vi "Custom Standard.vi"(0 "IL Enable":bool=TRUE, 5 "RL Enable":bool=TRUE) -> (7 "Output Custom":T1)   [LabVIEW 2017]
panel:
  in  "Min RL to Pass (dB)":dbl format="%#.2g"
  in  "Max IL to Pass (dB)":dbl=99.0 format="%.2g"
  in  "End Process":bool
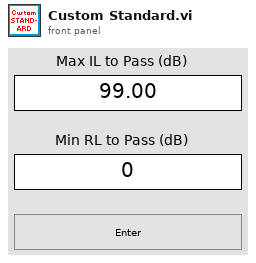
[diagram p1: front panel]
types:
  T1 = cluster{"Standard Name":string, "Max IL to Pass (dB)":dbl, "Min RL to Pass (dB)":dbl}
  T2 = enum8{"Enabled", "Disabled", "Disabled and Grayed Out"}
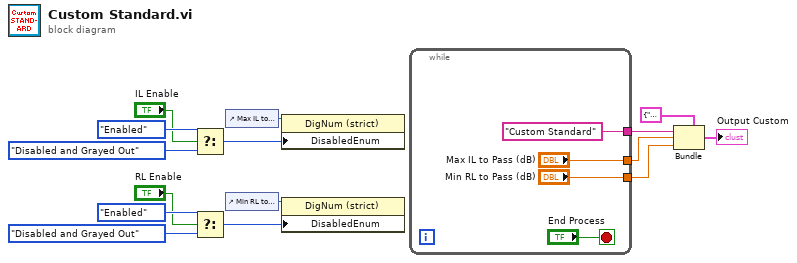
[diagram p0: block diagram]
diagram:
  n1 = Select(t=T2."Enabled" ("Disabled"), s="IL Enable", f=T2."Disabled and Grayed Out" ("Disabled")) -> (s? t:f=w6:T2)
  n2 = Select(t=T2."Enabled" ("Disabled"), s="RL Enable", f=T2."Disabled and Grayed Out" ("Disabled")) -> (s? t:f=w5:T2)
  n3 = control-ref of="Max IL to Pass (dB)"() -> (w10:refnum<vi>)
  n4 = control-ref of="Min RL to Pass (dB)"() -> (w9:refnum<vi>)
  n5 = property class="DigNum (strict)"(reference=w10, "DisabledEnum"=w6) -> ()  [unwired: 1 in, 2 out]
  n6 = property class="DigNum (strict)"(reference=w9, "DisabledEnum"=w5) -> ()  [unwired: 1 in, 2 out]
  n7 = while {
    tunnel: ["Custom Standard"] -> w14
    tunnel: ["Min RL to Pass (dB)"] -> w13
    tunnel: ["Max IL to Pass (dB)"] -> w12
    stop <- "End Process" stop-if-true
  }
  n8 = Bundle(cluster=T1 {"Standard Name"="", "Max IL to Pass (dB)"=0.0, "Min RL to Pass (dB)"=0.0} ("IL RL Standards"), "Standard Name"=w14, "Max IL to Pass (dB)"=w12, "Min RL to Pass (dB)"=w13) -> (→"Output Custom":T1)
